vi "INI-W-R.vi"(7 "W/R":enum16{"读", "写"}(ring)=enum."写", 11 "VI ref":refnum<vi>) -> (0 "error out":errorcluster)   [LabVIEW 2014]
uses:
  <vilib>/Utility/config.llb/NI_LVConfig.lvlib
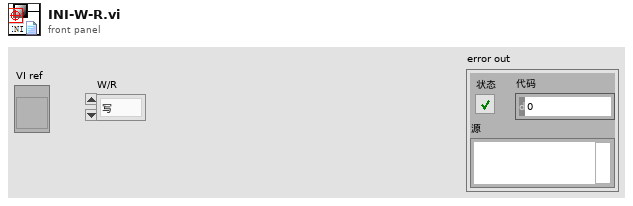
[diagram p1: front panel]
types:
  T1 = typedef "NI_LVConfig.lvlib/Config Data RefNum.ctl" = refnum<k1>
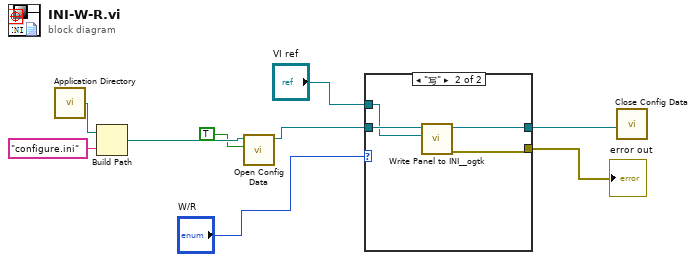
[diagram p0: block diagram]
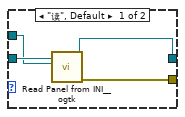
[diagram p2: hidden frame]
diagram:
  n1 = call <vilib>:"Application Directory.vi"() -> ("Application Directory"=w8:path)
  n2 = Build Path(base path=w8, name or relative path="configure.ini" ("名称或相对路径")) -> (appended path=w6:path)
  n3 = call <vilib>:"Open Config Data.vi"("create file if necessary (T)"=TRUE, "configuration file path"=w6) -> ("refnum"=w9:T1)  [unwired: 7 in, 2 out]
  n4 = case shown="\"写\"" "W/R" {
    tunnel: w9 -> [w13 w17]
    tunnel: [w12 w16] -> w4
    tunnel: "VI ref" -> [w11 w15]
    tunnel: [w10 w14] -> w1
    frame "读", Default {
      n5 = call "Read Panel from INI__ogtk.vi"("VI ref"=w11, "refnum"=w13) -> ("error out"=w10:errorcluster, "refnum out"=w12:T1)  [unwired: 8 in]
    }
    frame "写" {
      n6 = call "Write Panel to INI__ogtk.vi"("VI ref"=w15, "refnum"=w17) -> ("error out"=w14:errorcluster, "refnum out"=w16:T1)  [unwired: 8 in]
    }
  }
  "error out" <- w1
  n7 = call <vilib>:"Close Config Data.vi"("refnum"=w4) -> ()  [unwired: 9 in, 2 out]
